vi "Read Value.vi"(8 "Error In":errorcluster, 11 "Pair In":refnum<class "Pair.lvclass">) -> (0 "Error Out":errorcluster, 2 "Value":refnum<class "Datum.lvclass">, 3 "Pair Out":refnum<class "Pair.lvclass">)   [LabVIEW 2018, in "Toolkit.lvlib" / "Data.lvlib" / "Pair.lvclass"]
doc: "Gets the Mustache value from the key-value pair.\n\n<B>Pair In/Out</B> - Represents a Mustache key-value pair.\n\n<B>Value</B> - Represents a Mustache value from the key-value pair."
uses:
  Pair.lvclass
  Datum/Datum.lvclass
  Pair.lvclass/Pair.ctl
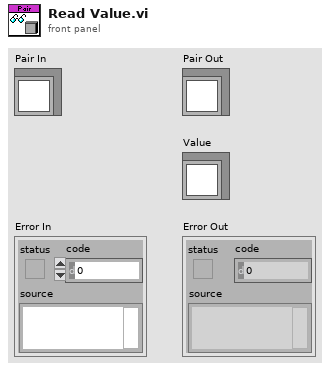
[diagram p1: front panel]
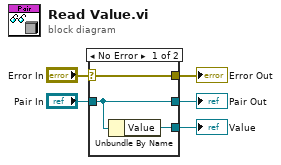
[diagram p0: block diagram]
diagram:
  n1 = case shown="No Error" "Error In" {
    selector: "Error In" -> [w8 w9]
    tunnel: [w8 w9] -> w4
    tunnel: [w7 w10] -> w2
    tunnel: "Pair In" -> [w7 w10]
    tunnel: [w6 _] -> w1
    frame No Error {
      n2 = Unbundle By Name(w7) -> ("Value"=w6:refnum<class "Datum.lvclass">)
    }
    frame Error {
    }
  }
  "Error Out" <- w4
  "Pair Out" <- w2
  "Value" <- w1
